vi "set ABS (SubVI).vi"(1 "En":bool, 2 "in":dbl) -> (6 "out":dbl)   [LabVIEW 2015]
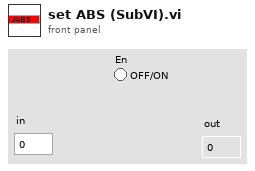
[diagram p1: front panel]
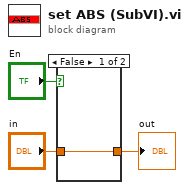
[diagram p0: block diagram]
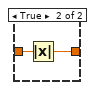
[diagram p2: hidden frame]
diagram:
  n1 = case shown="False" "En" {
    tunnel: "in" -> [w4 w6]
    tunnel: [w4 w5] -> w2
    frame False {
    }
    frame True {
      n2 = Absolute Value(x=w6) -> (abs(x)=w5:dbl)
    }
  }
  "out" <- w2
